vi "LoadSequence.vi"(8 "error in (no error)":errorcluster, 9 "Sequence Cfg":T2, 10 "Message que":T1, 11 "Sequence in":refnum<class "Sequence.lvclass">) -> (0 "error out":errorcluster, 3 "Sequence out":refnum<class "Sequence.lvclass">)   [LabVIEW 2019, in "Sequence.lvclass"]
uses:
  Sequence.lvclass
  seqConfig.ctl
  Support/MessageQue/MessageQue.ctl
  Support/MessageQue/MessageCluster.ctl
  SendMessage/SendMessage.lvclass
  SequenceSubvis/mWaveTestStep.ctl
  SequenceSubvis/TestStepTypes.ctl
  SequenceSubvis/RF Direction.ctl
  SequenceSubvis/PolarizationSelect.ctl
  APARMainSubvis/VXM Public API/singleAxisMoveDef.ctl
  APARMainSubvis/VXM Public API/mmWaveAxis.ctl
  Sequence.lvclass/Sequence.ctl
  Support/MessageQue/MessageQue.lvlib
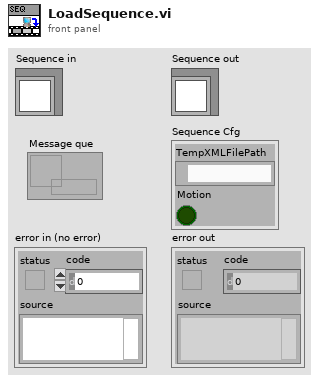
[diagram p1: front panel]
types:
  T1 = typedef "MessageQue.lvlib/MessageQue.ctl" = refnum<queue>
  T2 = typedef "seqConfig.ctl" = cluster{"TempXMLFilePath":path, "Motion":bool}
  T3 = typedef "mWaveTestStep.ctl" = cluster{"StepType":T4, "RF In/Out":T5, "Module/Raster":i32, "Polarization":T6, "AO-64 Array":dbl[], "Position":T7[]}
  T4 = typedef "TestStepTypes.ctl" = enum16{"MotionFF-M2", "Motion", "SweepTest", "RasterTest", "Finish", "64ModuleCfg"}
  T5 = typedef "RF Direction.ctl" = enum16{"Tx - RF In", "Rx - RF Out"}
  T6 = typedef "PolarizationSelect.ctl" = enum16{"Vertical", "Horizontal"}
  T7 = typedef "singleAxisMoveDef.ctl" = cluster{"mmWave Axis":T8, "eng. value":dbl}
  T8 = typedef "mmWaveAxis.ctl" = string
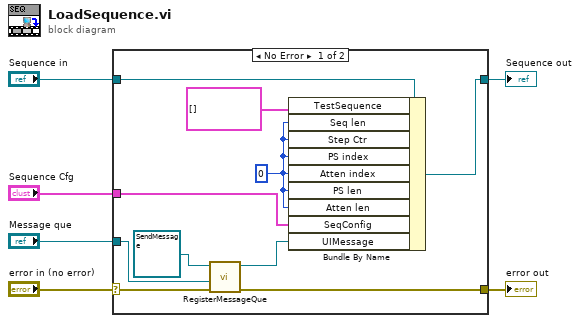
[diagram p0: block diagram]
diagram:
  n1 = case shown="No Error" "error in (no error)" {
    selector: "error in (no error)" -> [w10 w18]
    tunnel: [w7 w18] -> w5
    tunnel: [w8 w17] -> w3
    tunnel: "Sequence in" -> [w16 w17]
    tunnel: "Sequence Cfg" -> [w14 _]
    tunnel: "Message que" -> [w12 _]
    frame No Error {
      w15 = 0 ("Execution.Step Ctr")
      n2 = call "RegisterMessageQue.vi"("error in (no error)"=w10, "Message que"=w12, "SendMessage in"=refnum<class "SendMessage.lvclass"> refnum) -> ("error out"=w7:errorcluster, "SendMessage out"=w13:refnum<class "SendMessage.lvclass">)  [unwired: 7 in]
      n3 = Bundle By Name(cluster=w16, "TestSequence"=T3[] [], "Seq len"=w15, "Step Ctr"=w15, "PS index"=w15, "Atten index"=w15, "PS len"=w15, "Atten len"=w15, "SeqConfig"=w14, "UIMessage"=w13) -> (w8:refnum<class "Sequence.lvclass">)
    }
    frame Error {
    }
  }
  "error out" <- w5
  "Sequence out" <- w3
